vi "Write_Spreadsheet.vi"(10 "Data In":T2, 11 "Data":T1) -> ()   [LabVIEW 2017]
doc: "SubVI que ayuda a actualizar el Spreadsheet dependiendo de que es lo que se desea actualizar."
uses:
  Controls/Data_In.ctl
  Controls/Data.ctl
  <vilib>/Utility/file.llb/Read Delimited Spreadsheet (string).vi
  <vilib>/Utility/file.llb/Write Delimited Spreadsheet (string).vi
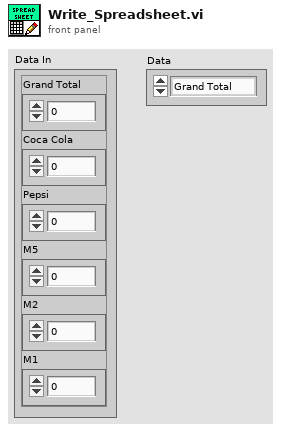
[diagram p1: front panel]
types:
  T1 = typedef "Data.ctl" = enum16{"Grand Total", "Coca-Cola", "Pepsi", "M1", "M2", "M5"}
  T2 = typedef "Data_In.ctl" = cluster{"Grand Total":i32, "Coca Cola":i32, "Pepsi":i32, "M5":i32, "M2":i32, "M1":i32}
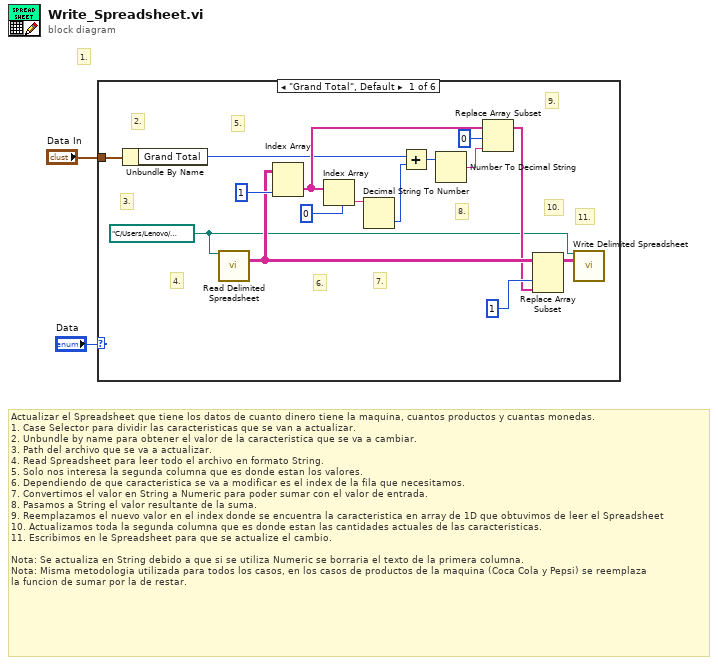
[diagram p0: block diagram]
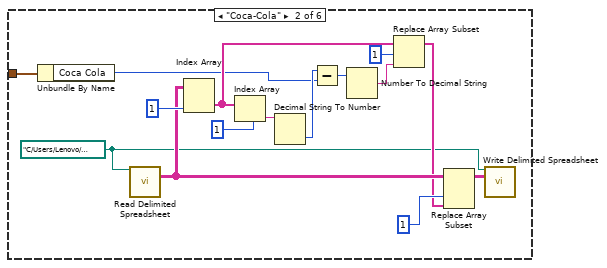
[diagram p2: hidden frame]
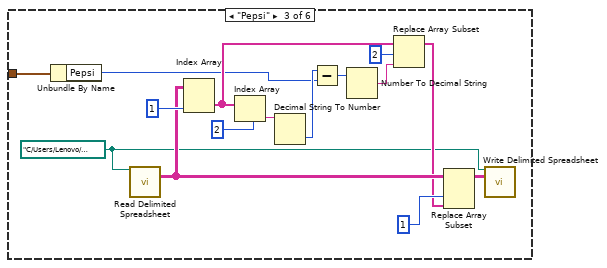
[diagram p3: hidden frame]
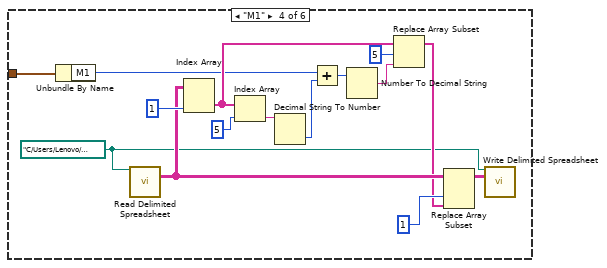
[diagram p4: hidden frame]
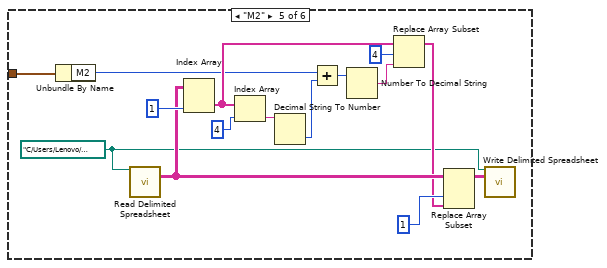
[diagram p5: hidden frame]
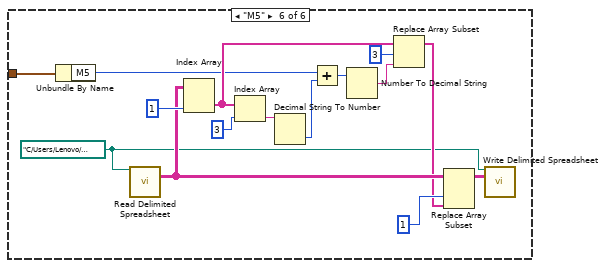
[diagram p6: hidden frame]
diagram:
  # "Actualizar el Spreadsheet que tiene los datos de cuanto dinero tiene la maquina, cuantos productos y cuantas monedas.\n1. Case Selector para dividir las caracteristicas que se van a actualizar.\n2. Unbundle by name para obtener el valor de la caracteristica que se va a cambiar.\n3. Path del archivo que se va a actualizar.\n4. Read Spreadsheet para leer todo el archivo en formato String.\n5. Solo nos interesa la segunda columna que es donde estan los valores.\n6. Dependiendo de que caracteristica se va a modificar es el index de la fila que necesitamos.\n7. Convertimos el valor en String a Numeric para poder sumar con el valor de entrada.\n8. Pasamos a String el valor resultante de la suma.\n9. Reemplazamos el nuevo valor en el index donde se encuentra la caracteristica en array de 1D que obtuvimos de leer el Spreadsheet\n10. Actualizamos toda la segunda columna que es donde estan las cantidades actuales de las caracteristicas.\n11. Escribimos en le Spreadsheet para que se actualize el cambio.\n\nNota: Se actualiza en String debido a que si se utiliza Numeric se borraria el texto de la primera columna.\nNota: Misma metodologia utilizada para todos los casos, en los casos de productos de la maquina (Coca Cola y Pepsi) se reemplaza\nla funcion de sumar por la de restar."
  # "1."
  n1 = case shown="\"Grand Total\", Default" "Data" {
    tunnel: "Data In" -> [w17 w32 w47 w62 w77 w92]
    frame "Grand Total", Default {
      w10 = path "C:/Users/Lenovo/Google Drive/Labview/Curso (FIME)/HW/Act. 3/HW. 3/Stuff/Data.txt" ("file path (dialog if empty)")
      # "11."
      # "10."
      # "9."
      # "8."
      # "7."
      # "6."
      # "5."
      # "4."
      # "3."
      # "2."
      n2 = Unbundle By Name(w17) -> ("Grand Total"=w5:i32)
      n3 = call-poly <vilib>:"Read Delimited Spreadsheet.vi"("file path (dialog if empty)"=w10) -> ("all rows"=w14:string[][])  [unwired: 9 in, 5 out]
      n4 = Index Array(array=w14, index (col)=1 ("disabled index (col)")) -> (element=w9:string[])  [unwired: 1 in]
      n5 = Index Array(array=w9, index=0) -> (element=w7:string)
      n6 = Decimal String To Number(string=w7) -> (number=w6:i32)  [unwired: 2 in, 1 out]
      n7 = Add(x=w5, y=w6) -> (x+y=w4:i32)
      n8 = Number To Decimal String(number=w4) -> (decimal integer string=w3:string)  [unwired: 1 in]
      n9 = Replace Array Subset(array=w9, new element=w3, index=0) -> (w12:string[])
      n10 = Replace Array Subset(array=w14, new element=w12, index (col)=1 ("disabled index (col)")) -> (w11:string[][])  [unwired: 1 in]
      n11 = call-poly <vilib>:"Write Delimited Spreadsheet.vi"("file path (dialog if empty)"=w10, "2D data"=w11) -> ()  [unwired: 12 in, 2 out]
    }
    frame "Coca-Cola" {
      w25 = path "C:/Users/Lenovo/Google Drive/Labview/Curso (FIME)/HW/Act. 3/HW. 3/Stuff/Data.txt" ("file path (dialog if empty)")
      n12 = Unbundle By Name(w32) -> ("Coca Cola"=w18:i32)
      n13 = call-poly <vilib>:"Read Delimited Spreadsheet.vi"("file path (dialog if empty)"=w25) -> ("all rows"=w29:string[][])  [unwired: 9 in, 5 out]
      n14 = Index Array(array=w29, index (col)=1 ("disabled index (col)")) -> (element=w24:string[])  [unwired: 1 in]
      n15 = Index Array(array=w24, index=1) -> (element=w22:string)
      n16 = Decimal String To Number(string=w22) -> (number=w19:i32)  [unwired: 2 in, 1 out]
      n17 = Subtract(x=w19, y=w18) -> (x-y=w21:i32)
      n18 = Number To Decimal String(number=w21) -> (decimal integer string=w20:string)  [unwired: 1 in]
      n19 = Replace Array Subset(array=w24, new element=w20, index=1) -> (w27:string[])
      n20 = Replace Array Subset(array=w29, new element=w27, index (col)=1 ("disabled index (col)")) -> (w26:string[][])  [unwired: 1 in]
      n21 = call-poly <vilib>:"Write Delimited Spreadsheet.vi"("file path (dialog if empty)"=w25, "2D data"=w26) -> ()  [unwired: 12 in, 2 out]
    }
    frame "Pepsi" {
      w40 = path "C:/Users/Lenovo/Google Drive/Labview/Curso (FIME)/HW/Act. 3/HW. 3/Stuff/Data.txt" ("file path (dialog if empty)")
      n22 = Unbundle By Name(w47) -> ("Pepsi"=w33:i32)
      n23 = call-poly <vilib>:"Read Delimited Spreadsheet.vi"("file path (dialog if empty)"=w40) -> ("all rows"=w44:string[][])  [unwired: 9 in, 5 out]
      n24 = Index Array(array=w44, index (col)=1 ("disabled index (col)")) -> (element=w39:string[])  [unwired: 1 in]
      n25 = Index Array(array=w39, index=2) -> (element=w37:string)
      n26 = Decimal String To Number(string=w37) -> (number=w34:i32)  [unwired: 2 in, 1 out]
      n27 = Subtract(x=w34, y=w33) -> (x-y=w36:i32)
      n28 = Number To Decimal String(number=w36) -> (decimal integer string=w35:string)  [unwired: 1 in]
      n29 = Replace Array Subset(array=w39, new element=w35, index=2) -> (w42:string[])
      n30 = Replace Array Subset(array=w44, new element=w42, index (col)=1 ("disabled index (col)")) -> (w41:string[][])  [unwired: 1 in]
      n31 = call-poly <vilib>:"Write Delimited Spreadsheet.vi"("file path (dialog if empty)"=w40, "2D data"=w41) -> ()  [unwired: 12 in, 2 out]
    }
    frame "M1" {
      w55 = path "C:/Users/Lenovo/Google Drive/Labview/Curso (FIME)/HW/Act. 3/HW. 3/Stuff/Data.txt" ("file path (dialog if empty)")
      n32 = Unbundle By Name(w62) -> ("M1"=w50:i32)
      n33 = call-poly <vilib>:"Read Delimited Spreadsheet.vi"("file path (dialog if empty)"=w55) -> ("all rows"=w59:string[][])  [unwired: 9 in, 5 out]
      n34 = Index Array(array=w59, index (col)=1 ("disabled index (col)")) -> (element=w54:string[])  [unwired: 1 in]
      n35 = Index Array(array=w54, index=5) -> (element=w52:string)
      n36 = Decimal String To Number(string=w52) -> (number=w51:i32)  [unwired: 2 in, 1 out]
      n37 = Add(x=w50, y=w51) -> (x+y=w49:i32)
      n38 = Number To Decimal String(number=w49) -> (decimal integer string=w48:string)  [unwired: 1 in]
      n39 = Replace Array Subset(array=w54, new element=w48, index=5) -> (w57:string[])
      n40 = Replace Array Subset(array=w59, new element=w57, index (col)=1 ("disabled index (col)")) -> (w56:string[][])  [unwired: 1 in]
      n41 = call-poly <vilib>:"Write Delimited Spreadsheet.vi"("file path (dialog if empty)"=w55, "2D data"=w56) -> ()  [unwired: 12 in, 2 out]
    }
    frame "M2" {
      w70 = path "C:/Users/Lenovo/Google Drive/Labview/Curso (FIME)/HW/Act. 3/HW. 3/Stuff/Data.txt" ("file path (dialog if empty)")
      n42 = Unbundle By Name(w77) -> ("M2"=w65:i32)
      n43 = call-poly <vilib>:"Read Delimited Spreadsheet.vi"("file path (dialog if empty)"=w70) -> ("all rows"=w74:string[][])  [unwired: 9 in, 5 out]
      n44 = Index Array(array=w74, index (col)=1 ("disabled index (col)")) -> (element=w69:string[])  [unwired: 1 in]
      n45 = Index Array(array=w69, index=4) -> (element=w67:string)
      n46 = Decimal String To Number(string=w67) -> (number=w66:i32)  [unwired: 2 in, 1 out]
      n47 = Add(x=w65, y=w66) -> (x+y=w64:i32)
      n48 = Number To Decimal String(number=w64) -> (decimal integer string=w63:string)  [unwired: 1 in]
      n49 = Replace Array Subset(array=w69, new element=w63, index=4) -> (w72:string[])
      n50 = Replace Array Subset(array=w74, new element=w72, index (col)=1 ("disabled index (col)")) -> (w71:string[][])  [unwired: 1 in]
      n51 = call-poly <vilib>:"Write Delimited Spreadsheet.vi"("file path (dialog if empty)"=w70, "2D data"=w71) -> ()  [unwired: 12 in, 2 out]
    }
    frame "M5" {
      w85 = path "C:/Users/Lenovo/Google Drive/Labview/Curso (FIME)/HW/Act. 3/HW. 3/Stuff/Data.txt" ("file path (dialog if empty)")
      n52 = Unbundle By Name(w92) -> ("M5"=w80:i32)
      n53 = call-poly <vilib>:"Read Delimited Spreadsheet.vi"("file path (dialog if empty)"=w85) -> ("all rows"=w89:string[][])  [unwired: 9 in, 5 out]
      n54 = Index Array(array=w89, index (col)=1 ("disabled index (col)")) -> (element=w84:string[])  [unwired: 1 in]
      n55 = Index Array(array=w84, index=3) -> (element=w82:string)
      n56 = Decimal String To Number(string=w82) -> (number=w81:i32)  [unwired: 2 in, 1 out]
      n57 = Add(x=w80, y=w81) -> (x+y=w79:i32)
      n58 = Number To Decimal String(number=w79) -> (decimal integer string=w78:string)  [unwired: 1 in]
      n59 = Replace Array Subset(array=w84, new element=w78, index=3) -> (w87:string[])
      n60 = Replace Array Subset(array=w89, new element=w87, index (col)=1 ("disabled index (col)")) -> (w86:string[][])  [unwired: 1 in]
      n61 = call-poly <vilib>:"Write Delimited Spreadsheet.vi"("file path (dialog if empty)"=w85, "2D data"=w86) -> ()  [unwired: 12 in, 2 out]
    }
  }
